vi "PTSequencer.index DIM subscriptions.vi"(0 "i ref in":refnum<vi>, 3 "ms timeout (10000)":i32=10000, 5 "error in":errorcluster) -> (14 "i ref out":refnum<vi>, 17 "timed out":bool, 19 "error out":errorcluster)   [LabVIEW 2014, in "PTSequencer.lvlib"]
uses:
  PTSequencer.lvlib
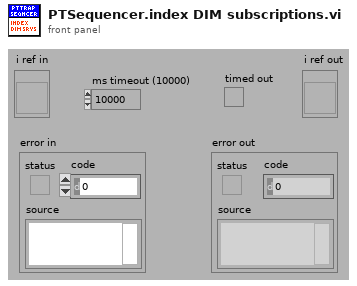
[diagram p1: front panel]
types:
  T1 = cluster{"step condition IDs":cluster{"step ID":i32, "condition ID":i32}[]}[]
  T2 = typedef "PTSequencer.lvlib/PTSequencer.i attribute.ctl" = cluster{"subsequence":bool, "mode":T3, "i step":i32, "nofLoops":i32, "i loop":i32, "Running":bool, "Paused":bool, "step done":bool, "loop done":bool, "seq done":bool, "DIM IDs":cluster{"step done":i32, "loop done":i32, "seq done":i32, "i step":i32, "i loop":i32}, "use stop conditions":bool, "stop conditions":T4[], "Step List":T6[], "DIM subsriptions":string[], "stop cond indexes":i32[], "step cond indexes":cluster{"step condition IDs":cluster{"step ID":i32, "condition ID":i32}[]}[], "Delay Start Time":timestamp, "status":string, "stopping":bool}
  T3 = typedef "PTSequencer.lvlib/PTSequencer.mode.ctl" = enum16{"single", "loop", "for loop"}
  T4 = typedef "PTSequencer.lvlib/PTSequencer.DIM service condition.ctl" = cluster{"DIM service":string, "descr":string, "nomValue":T5, "actValue":T5, "matched":bool, "DIM Status":cluster{"no link":bool, "quality":i32, "Time Stamp":timestamp}}
  T5 = typedef "CoreDefs.rawDataType.ctl" = i8[]
  T6 = typedef "PTSequencer.lvlib/PTSequencer.step.ctl" = cluster{"description":string, "object parameters":cluster{"object":string, "selector":string, "descriptor":string, "data":T5, "subsequence":bool, "call mode":enum16{"Simple DIM", "Synchronous"}, "data in":T5}, "result action":cluster{"check":bool, "passed":enum16{"Next", "Previous", "Repeat", "Jump"}, "failed":enum16{"Next", "Previous", "Repeat", "Jump"}, "jumpID_passed":i32, "jumpID_failed":i32}, "conditions":T4[], "fulfilled ":bool, "use delay":bool, "delay time (s)":dbl, "ID":i32}
  T7 = cluster{"step condition IDs":cluster{"step ID":i32, "condition ID":i32}[]}
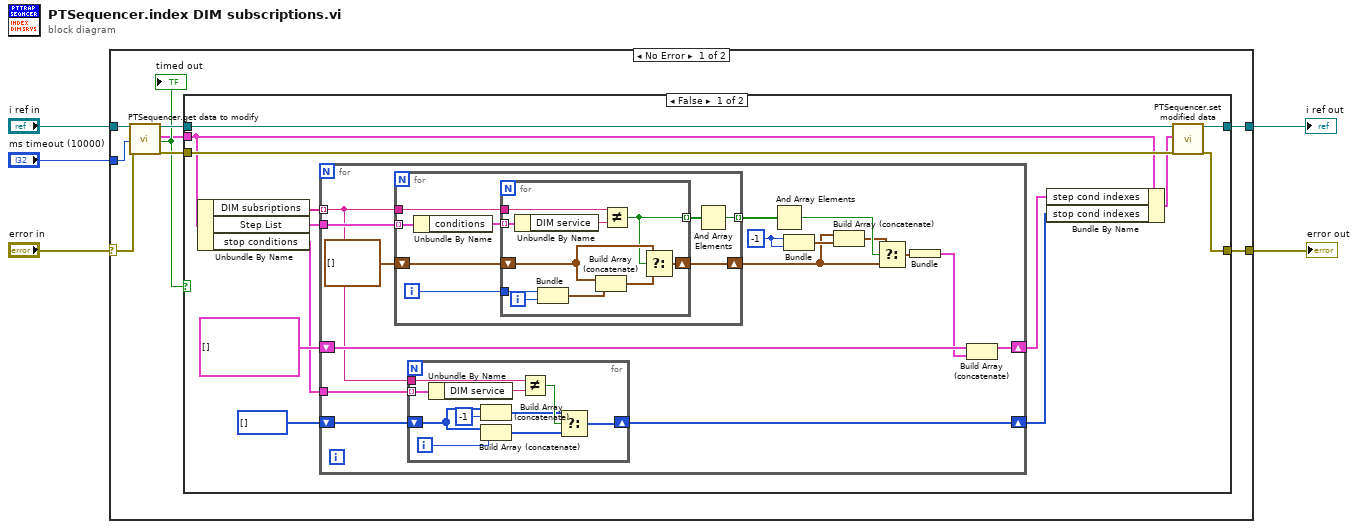
[diagram p0: block diagram]
diagram:
  n1 = case shown="No Error" "error in" {
    selector: "error in" -> [w12 w74]
    tunnel: "i ref in" -> [w9 w75]
    tunnel: [w14 w75] -> w4
    tunnel: [w13 w74] -> w3
    tunnel: "ms timeout (10000)" -> [w6 _]
    frame No Error {
      n2 = call "PTSequencer.get data to modify.vi"("i ref in"=w9, "ms timeout (10000)"=w6, "error in (no error)"=w12) -> ("i ref out"=w10:refnum<vi>, "i attribute"=w7:T2, "timed out"=w8:bool, "error out"=w11:errorcluster)  [unwired: 13 in]
      "timed out" <- w8
      n3 = case shown="False" w8 {
        tunnel: [w23 w72] -> w14
        tunnel: [w19 w73] -> w13
        tunnel: w11 -> [w26 w73]
        tunnel: w10 -> [w27 w72]
        tunnel: w7 -> [w24 _]
        frame False {
          n4 = Unbundle By Name(w24) -> ("DIM subsriptions"=w22:string[], "Step List"=w18:T6[], "stop conditions"=w17:T4[])
          n5 = for {
            tunnel: w22 -> [w37] mode=indexing
            shift-right: [w40] -> w16
            shift-left: T1 [] ("step cond indexes") -> [w41]
            shift-right: [w35] -> w15
            shift-left: i32[] [] -> [w36]
            tunnel: w18 -> [w43]
            tunnel: w17 -> [w38]
            w28 = -1
            n6 = for {
              tunnel: w43 -> [w61] mode=indexing
              shift-right: [w56] -> w29
              shift-left: cluster{"step ID":i32, "condition ID":i32}[] [] ("step condition IDs") -> [w59]
              tunnel: w37 -> [w58]
              tunnel: [w54] -> w34 mode=indexing
              i -> [w57]
              n7 = Unbundle By Name(w61) -> ("conditions"=w60:T4[])
              n8 = for {
                tunnel: w60 -> [w70] mode=indexing
                shift-right: [w65] -> w56
                shift-left: w59 -> [w63]
                tunnel: w58 -> [w71]
                tunnel: w57 -> [w68]
                tunnel: [w62] -> w55 mode=indexing
                i -> [w67]
                n9 = Unbundle By Name(w70) -> ("DIM service"=w69:string)
                n10 = Bundle(w68, w67) -> (w66:cluster{i32, i32})  [unwired: 1 in]
                n11 = Build Array (concatenate)(w63, w66) -> (w64:cluster{"step ID":i32, "condition ID":i32}[])
                n12 = Not Equal?(x=w71, y=w69) -> (x != y?=w62:bool)
                n13 = Select(t=w63, s=w62, f=w64) -> (s? t:f=w65:cluster{"step ID":i32, "condition ID":i32}[])
              }
              n14 = And Array Elements(Boolean array=w55) -> (logical AND=w54:bool)
            }
            n15 = for {
              tunnel: w38 -> [w53] mode=indexing
              tunnel: w37 -> [w52]
              shift-right: [w49] -> w35
              shift-left: w36 -> [w46]
              i -> [w48]
              n16 = Unbundle By Name(w53) -> ("DIM service"=w51:string)
              n17 = Build Array (concatenate)(w46, -1) -> (w45:i32[])
              n18 = Build Array (concatenate)(w46, w48) -> (w47:i32[])
              n19 = Not Equal?(x=w52, y=w51) -> (x != y?=w50:bool)
              n20 = Select(t=w45, s=w50, f=w47) -> (s? t:f=w49:i32[])
            }
            n21 = And Array Elements(Boolean array=w34) -> (logical AND=w33:bool)
            n22 = Bundle(w28, w28) -> (w32:cluster{i32, i32})  [unwired: 1 in]
            n23 = Build Array (concatenate)(w29, w32) -> (w31:cluster{"step ID":i32, "condition ID":i32}[])
            n24 = Select(t=w31, s=w33, f=w29) -> (s? t:f=w30:cluster{"step ID":i32, "condition ID":i32}[])
            n25 = Bundle("step condition IDs"=w30) -> (w39:T7)  [unwired: 1 in]
            n26 = Build Array (concatenate)(w41, w39) -> (w40:T1)
          }
          n27 = Bundle By Name(cluster=w24, "step cond indexes"=w16, "stop cond indexes"=w15) -> (w25:T2)
          n28 = call "PTSequencer.set modified data.vi"("i ref in"=w27, "CLASS.i attribute"=w25, "error in (no error)"=w26) -> ("i ref out"=w23:refnum<vi>, "error out"=w19:errorcluster)  [unwired: 15 in]
        }
        frame True {
        }
      }
    }
    frame Error {
    }
  }
  "i ref out" <- w4
  "error out" <- w3
